vi "validate configuration.vi"(8 "error in":errorcluster, 11 "sample module configuration in":refnum<class "sample module configuration.lvclass">) -> (0 "error out":errorcluster, 3 "sample module configuration out":refnum<class "sample module configuration.lvclass">)   [LabVIEW 2013, in "sample module configuration.lvclass"]
doc: "This function performs validation of the configuration. This function should be safe to call at any point and should not rely on anything in the runtime environment."
uses:
  sample module configuration.lvclass
  module configuration/TBM module configuration.lvclass
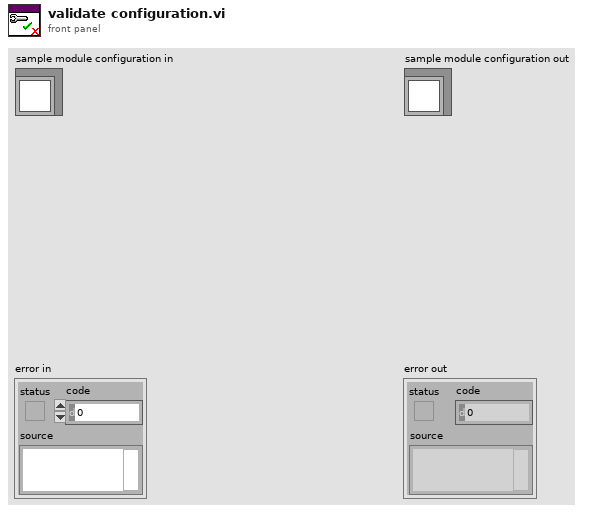
[diagram p1: front panel]
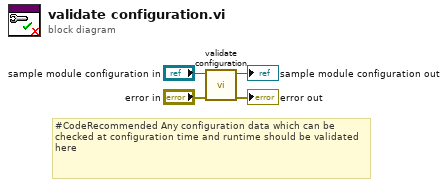
[diagram p0: block diagram]
diagram:
  # "#CodeRecommended Any configuration data which can be checked at configuration time and runtime should be validated here"
  n1 = call-parent "validate configuration.vi"("error in"="error in", "configuration in"="sample module configuration in") -> ("error out"=→"error out":errorcluster, "configuration out"=→"sample module configuration out":refnum<class "sample module configuration.lvclass">)  [unwired: 8 in]
